vi "JMP Im.vi"(8 "error in (no error)":errorcluster, 10 "Im":u8 format="%04b", 11 "TD4 in":refnum<class "TD4.lvclass">) -> (0 "error out":errorcluster, 3 "TD4 out":refnum<class "TD4.lvclass">)   [LabVIEW 2025, in "TD4.lvclass"]
uses:
  TD4.lvclass
  TD4.lvclass/TD4.ctl
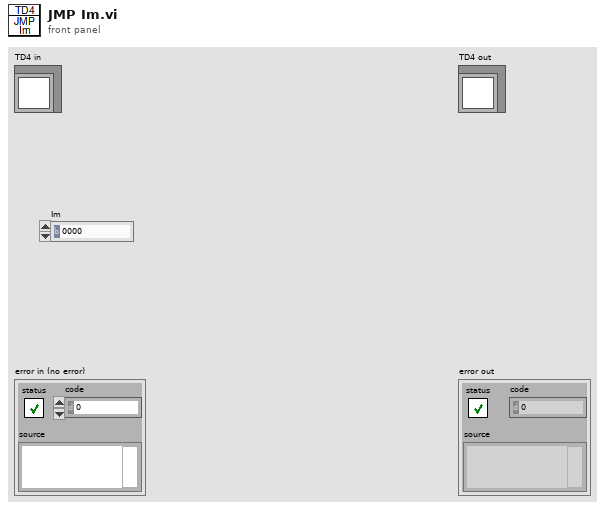
[diagram p1: front panel]
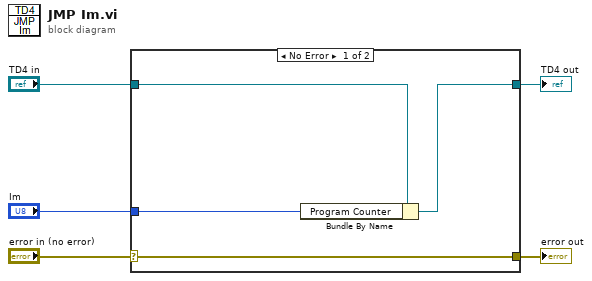
[diagram p0: block diagram]
diagram:
  n1 = case shown="No Error" "error in (no error)" {
    selector: "error in (no error)" -> [w9 w10]
    tunnel: [w9 w10] -> w4
    tunnel: [w7 w11] -> w2
    tunnel: "TD4 in" -> [w8 w11]
    tunnel: "Im" -> [w6 _]
    frame No Error {
      n2 = Bundle By Name(cluster=w8, "Program Counter"=w6) -> (w7:refnum<class "TD4.lvclass">)
    }
    frame Error {
    }
  }
  "error out" <- w4
  "TD4 out" <- w2
